vi "Field.vi"(1 "Action":T2=enum."Identify", 2 "Parameters":variant) -> (6 "Output":variant, 7 "Stop":bool)   [LabVIEW 2025]
doc: "Author: Scott Hannahs <sth@magnet.fsu.edu>\n\nThis software is licensed for use under the “MIT License\"\nCopyright (c) 2025 Scott Hannahs, sth@sth@magnet.sthnet.net\n\nPermission is hereby granted, free of charge, to any person obtaining a copy of this software and associated documentation files (the \"Software\"), to deal in the Software without restriction, including without limitation the rights to use, copy, modify, merge, publish, distribute, sublicense, and/or sell copies of the Software, and to permit persons to whom the Software is furnished to do so, subject to the following conditions: The above copyright notice and this permission notice shall be included in all copies or substantial portions of the Software.\n\nTHE SOFTWARE IS PROVIDED \"AS IS\", WITHOUT WARRANTY OF ANY KIND, EXPRESS OR IMPLIED, INCLUDING BUT NOT LIMITED TO THE WARRANTIES OF MERCHANTABILITY, FITNESS FOR A PARTICULAR PURPOSE AND NONINFRINGEMENT. IN NO EVENT SHALL THE AUTHORS OR COPYRIGHT HOLDERS BE LIABLE FOR ANY CLAIM, DAMAGES OR OTHER LIABILITY, WHETHER IN AN ACTION OF CONTRACT, TORT OR OTHERWISE, ARISING FROM, OUT OF OR IN CONNECTION WITH THE SOFTWARE OR THE USE OR OTHER DEALINGS IN THE SOFTWARE."
uses:
  Sub Controls/Instrument Actions.ctl
  Sub Controls/Public.ctl
  Sub Controls/User Event Command.ctl
  Sub Controls/Scan Output.ctl
panel:
  out "Title":string="Field"
  in  "Public":T1
  out "Measurement":dbl format="%.6f"
  in  "Field":bool=TRUE
  in  "Index":i32
  # "Current"
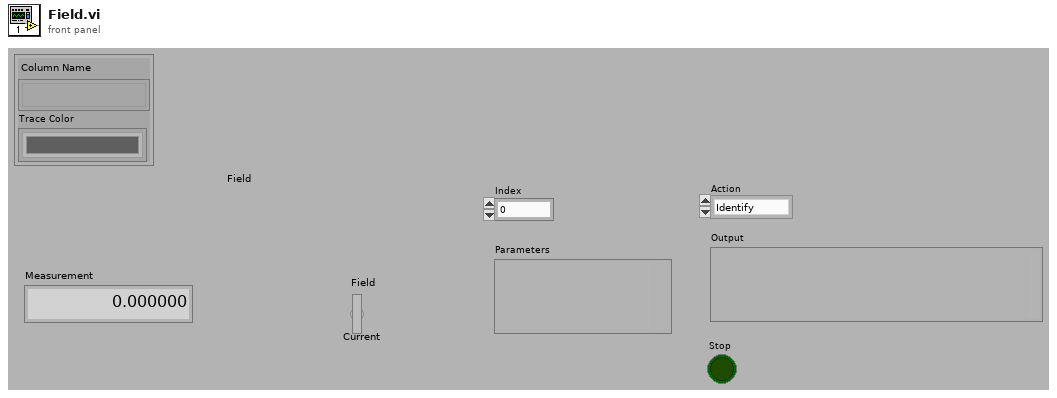
[diagram p1: front panel]
types:
  T1 = typedef "Public.ctl" = cluster{"Column Name":string[], "Trace Color":u32[]}
  T2 = typedef "Instrument Actions.ctl" = enum16{"Scan", "Identify", "New", "Configure", "Initialize", "Test", "Read", "Close"}
  T3 = typedef "User Event Command.ctl" = enum32{"Stop Config"}
  T4 = typedef "Scan Output.ctl" = cluster{"Manufacturer":string, "Model":string, "Info":string, "Revision":string, "error out":errorcluster}
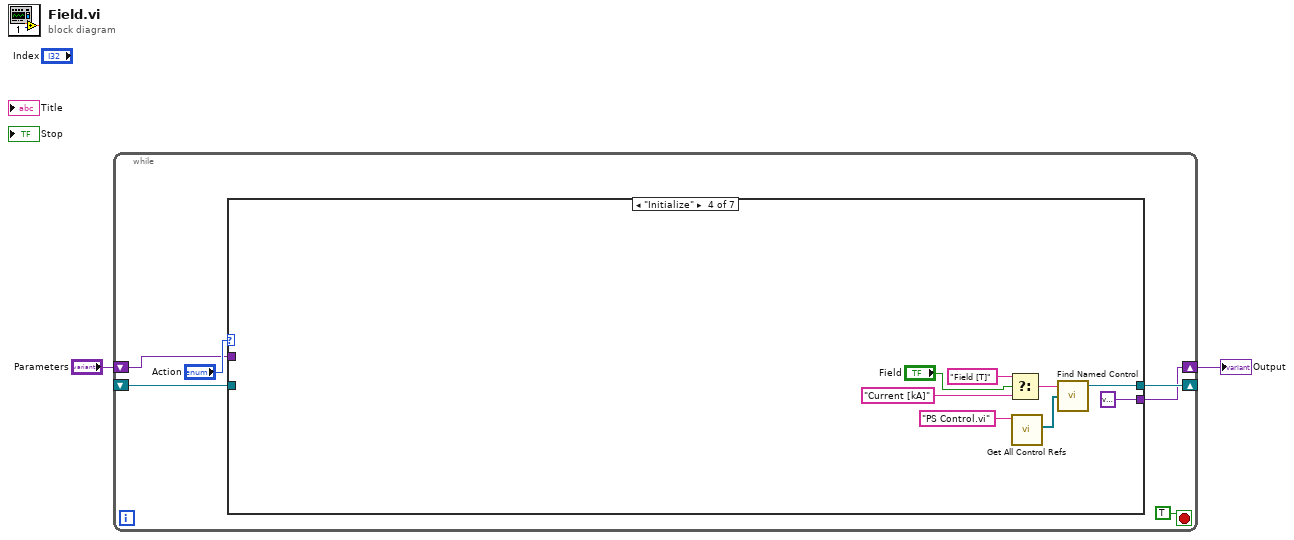
[diagram p0: block diagram]
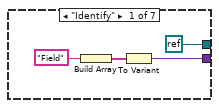
[diagram p2: hidden frame]
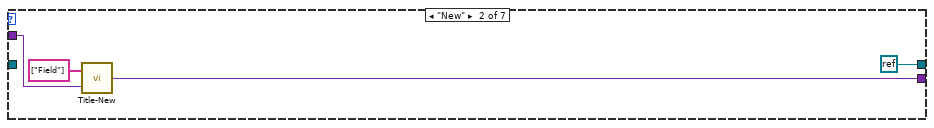
[diagram p3: hidden frame]
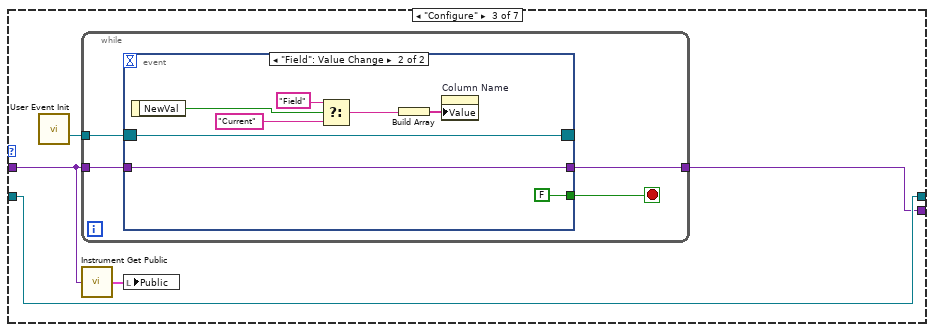
[diagram p4: hidden frame]
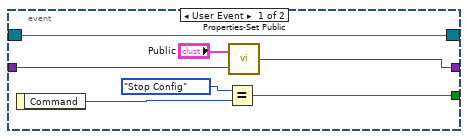
[diagram p5: hidden frame]
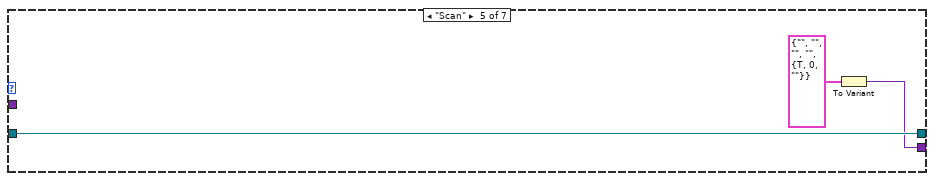
[diagram p6: hidden frame]
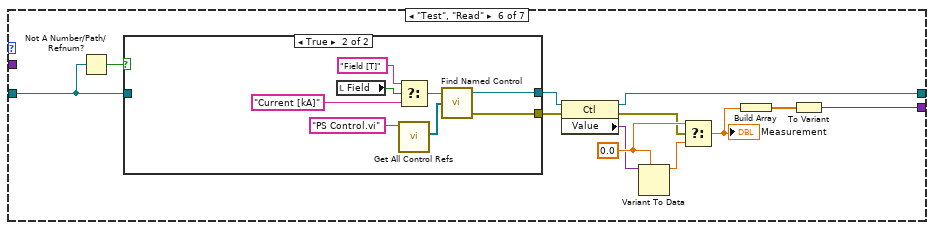
[diagram p7: hidden frame]
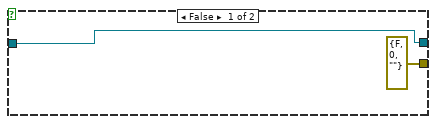
[diagram p8: hidden frame]
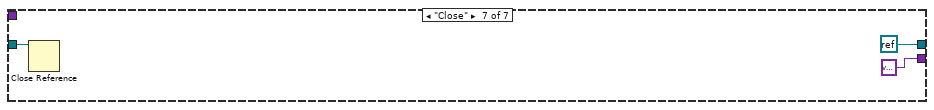
[diagram p9: hidden frame]
diagram:
  n1 = while {
    shift-right: [w7] -> _
    shift-left: _ -> [w6]
    shift-right: [w5] -> w2
    shift-left: "Parameters" -> [w4]
    stop <- TRUE stop-if-true
    n2 = case shown="\"Initialize\"" "Action" {
      tunnel: [w11 w15 w19 variant ("Variant") w50 w60 variant ("Variant")] -> w5
      tunnel: [refnum<k0> refnum refnum<k0> refnum w21 w42 w51 w55 refnum<k0> refnum] -> w7
      tunnel: w6 -> [_ _ w21 _ w51 w57 w76]
      tunnel: w4 -> [_ w14 w20 _ _ _ _]
      frame "Identify" {
        n3 = Build Array("Field") -> (w10:string[])
        n4 = To Variant(anything=w10) -> (Variant=w11:variant)
      }
      frame "New" {
        n5 = call "Title-New.vi"("Parameters"=w14, "Array"=string[] ["Field"]) -> ("Instrument Prop"=w15:variant)
      }
      frame "Configure" {
        n6 = call "User Event Init.vi"() -> ("Event Registration Refnum"=w17:refnum<event-registration>)  [unwired: 14 in, 1 out]
        n7 = while {
          tunnel: w20 -> [w25]
          tunnel: [w24] -> w19
          tunnel: w17 -> [w22]
          stop <- w23 stop-if-true
          n8 = event shown="[1] \"Field\": Value Change" {
            selector: w22 -> [w26 w33]
            dyn-events: [w26 w33] -> _
            timeout: _ -> [_ _]
            tunnel: [w32 w34] -> w24
            tunnel: [w28 FALSE ("NewVal")] -> w23
            tunnel: w25 -> [w31 w34]
            event User Event {
              n9 = event-data() -> ("Command"=w30:T3)  [unwired: 1 in]
              n10 = Equal?(x=User_Event_Command."Stop Config", y=w30) -> (x = y?=w28:bool)
              n11 = call "Properties-Set Public.vi"("Variant"=w31, "New Public"="Public") -> ("Variant 2"=w32:variant)
            }
            event "Field": Value Change {
              n12 = event-data() -> ("NewVal"=w40:bool)  [unwired: 1 in]
              n13 = Select(t="Field", s=w40, f="Current") -> (s? t:f=w39:string)
              n14 = Build Array(w39) -> (w35:string[])
              n15 = property on="Column Name" class="Arr (strict)"("Value"=w35) -> ()  [unwired: 2 in, 2 out]
            }
          }
        }
        n16 = call "Instrument Get Public.vi"("Variant"=w20) -> ("Public"=w18:T1)
        n17 = local write "Public"(w18) -> ()
      }
      frame "Initialize" {
        n18 = Select(t="Field [T]" ("Control Name"), s="Field", f="Current [kA]") -> (s? t:f=w43:string)
        n19 = call "Get All Control Refs.vi"("VI Name"="PS Control.vi") -> ("All Controls"=w46:refnum<vi>[])  [unwired: 5 in, 2 out]
        n20 = call "Find Named Control.vi"("All Controls"=w46, "Control Name"=w43) -> ("Ctl Refnum"=w42:refnum<vi>)  [unwired: 1 in, 2 out]
      }
      frame "Scan" {
        n21 = To Variant(anything=T4 {"Manufacturer"="", "Model"="", "Info"="", "Revision"="", "error out"={"status"=TRUE, "code"=0, "source"=""}} ("Scan Output")) -> (Variant=w50:variant)
      }
      frame "Test", "Read" {
        w62 = 0.0
        n22 = Not A Number/Path/Refnum?(number/path/refnum=w57) -> (NaN/Path/Refnum?=w58:bool)
        n23 = case shown="True" w58 {
          tunnel: [w65 w67] -> w56
          tunnel: w57 -> [w65 _]
          tunnel: [errorcluster {"status"=FALSE, "code"=0, "source"=""} ("error out") w66] -> w52
          frame False {
          }
          frame True {
            n24 = local read "Field"() -> (w68:bool)
            n25 = Select(t="Field [T]" ("Control Name"), s=w68, f="Current [kA]") -> (s? t:f=w69:string)
            n26 = call "Get All Control Refs.vi"("VI Name"="PS Control.vi") -> ("All Controls"=w72:refnum<vi>[])  [unwired: 5 in, 2 out]
            n27 = call "Find Named Control.vi"("All Controls"=w72, "Control Name"=w69) -> ("error out"=w66:errorcluster, "Ctl Refnum"=w67:refnum<vi>)  [unwired: 1 in, 1 out]
          }
        }
        n28 = property class="Ctl"(reference=w56, error in=w52) -> (reference out=w55:refnum<vi>, error out=w53:errorcluster, "Value"=w54:variant)
        n29 = Variant To Data(type=w62, Variant=w54) -> (data=w63:dbl)  [unwired: 1 in, 1 out]
        n30 = Select(t=w62, s=w53, f=w63) -> (s? t:f=w61:dbl)
        "Measurement" <- w61
        n31 = Build Array(w61) -> (w59:dbl[])
        n32 = To Variant(anything=w59) -> (Variant=w60:variant)
      }
      frame "Close" {
        n33 = Close Reference(reference=w76) -> ()  [unwired: 1 in, 1 out]
      }
    }
  }
  "Output" <- w2
